vi "Unflatten Inline Execution Units.vi"(8 "error in (no error)":errorcluster, 11 "Compiled Inline Execution Units":T4[](array[typedef]) {"Outgoing Data References"."Data Reference" format="%.0x"; "Incoming Data References" format="%.0x"}) -> (0 "error out":errorcluster, 3 "Inline Execution Units":T1[](array[typedef]) {"Outgoing Data References"."Data Reference" format="%.0x"; "Incoming Data References" format="%.0x"})   [LabVIEW 2020, in "AIM ARINC 429 Engine.lvlib" / "Custom Device.lvlib"]
uses:
  Custom Device.lvlib
  Inline Execution Unit Compiled Information.ctl
  <vilib>/NI VeriStand/Custom Device API/Data Reference.ctl
  <vilib>/NI VeriStand/Custom Device API/Block Data Reference.ctl
  Inline Execution Unit Runtime Information.ctl
  Interfaces/Execution Unit/Execution Unit.lvclass
  <vilib>/NI VeriStand/Custom Device API/Custom Device API.lvlib
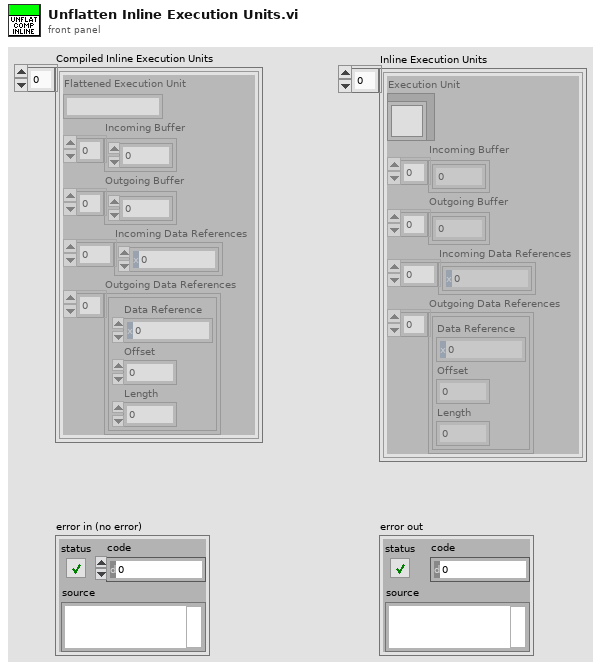
[diagram p1: front panel]
types:
  T1 = typedef "AIM ARINC 429 Engine.lvlib/Custom Device.lvlib/Inline Execution Unit Runtime Information.ctl" = cluster{"Execution Unit":refnum<class "Execution Unit.lvclass">, "Incoming Buffer":dbl[], "Outgoing Buffer":dbl[], "Incoming Data References":T2[], "Outgoing Data References":T3[]}
  T2 = typedef "Custom Device API.lvlib/Data Reference.ctl" = i32
  T3 = typedef "Custom Device API.lvlib/Block Data Reference.ctl" = cluster{"Data Reference":T2, "Offset":u64, "Length":u64}
  T4 = typedef "AIM ARINC 429 Engine.lvlib/Custom Device.lvlib/Inline Execution Unit Compiled Information.ctl" = cluster{"Flattened Execution Unit":string, "Incoming Buffer":dbl[], "Outgoing Buffer":dbl[], "Incoming Data References":T2[], "Outgoing Data References":T3[]}
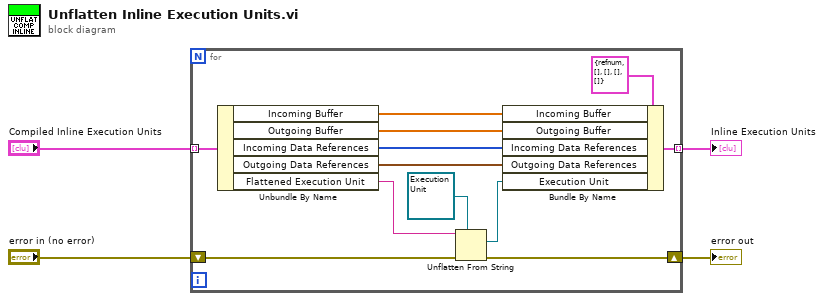
[diagram p0: block diagram]
diagram:
  n1 = for {
    tunnel: "Compiled Inline Execution Units" -> [w13] mode=indexing
    tunnel: [w9] -> w1 mode=indexing
    shift-right: [w15] -> w3
    shift-left: "error in (no error)" -> [w16]
    n2 = Unbundle By Name(w13) -> ("Incoming Buffer"=w8:dbl[], "Outgoing Buffer"=w7:dbl[], "Incoming Data References"=w6:T2[], "Outgoing Data References"=w5:T3[], "Flattened Execution Unit"=w10:string)
    n3 = Unflatten From String(type=refnum<class "Execution Unit.lvclass"> refnum ("Communication Bus Template Interfaces:Execution Unit.lvlib:Execution Unit.lvclass"), binary string=w10, error in (no error)=w16) -> (value=w11:refnum<class "Execution Unit.lvclass">, error out=w15:errorcluster)  [unwired: 2 in, 1 out]
    n4 = Bundle By Name(cluster=T1 {"Execution Unit"=refnum, "Incoming Buffer"=[], "Outgoing Buffer"=[], "Incoming Data References"=[], "Outgoing Data References"=[]} ("Inline Execution Unit Runtime Information"), "Incoming Buffer"=w8, "Outgoing Buffer"=w7, "Incoming Data References"=w6, "Outgoing Data References"=w5, "Execution Unit"=w11) -> (w9:T1)
  }
  "error out" <- w3
  "Inline Execution Units" <- w1
